vi "test Correct Subaddresses In Log.vi"(8 "error in (no error)":errorcluster, 11 "TestCase in":refnum<class "Logging Loopback.lvclass">) -> (0 "error out":errorcluster, 3 "TestCase out":refnum<class "Logging Loopback.lvclass">)   [LabVIEW 2020, in "Logging Loopback.lvclass"]
uses:
  Logging Loopback.lvclass
  Logging Loopback.lvclass/Logging Loopback.ctl
  6070ecc1-7a7f-4aba-84f3-8f274e3c644e.vi
  e19d9c75-8616-4056-a7e1-33fbf9884e17.vi
  <vilib>/WebDAVClient/Advanced/Get Buffer.vi
  <vilib>/addons/_JKI Toolkits/VI Tester/TestCase.llb/TestCase.lvclass
  <vilib>/WebDAVClient/NI_WebDAV.lvlib
  C:/Program Files (x86)/National Instruments/LabVIEW 2020/vi.lib/addons/_JKI Toolkits/VI Tester/TestCase.llb/TestCase.lvclass
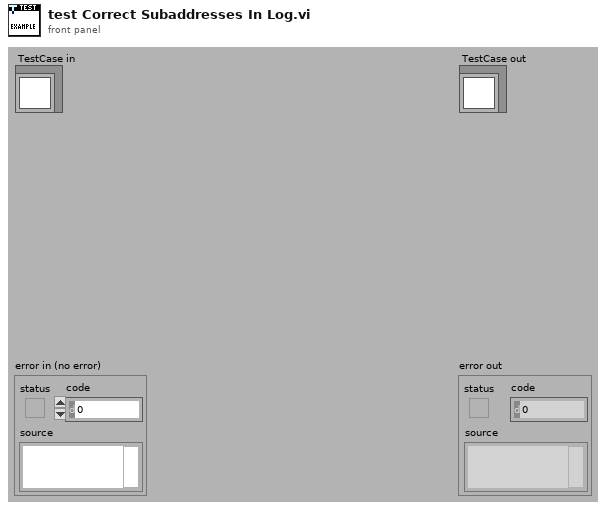
[diagram p1: front panel]
types:
  T1 = typedef "NI_WebDAV.lvlib/SessionHandle.ctl" = refnum<k1>
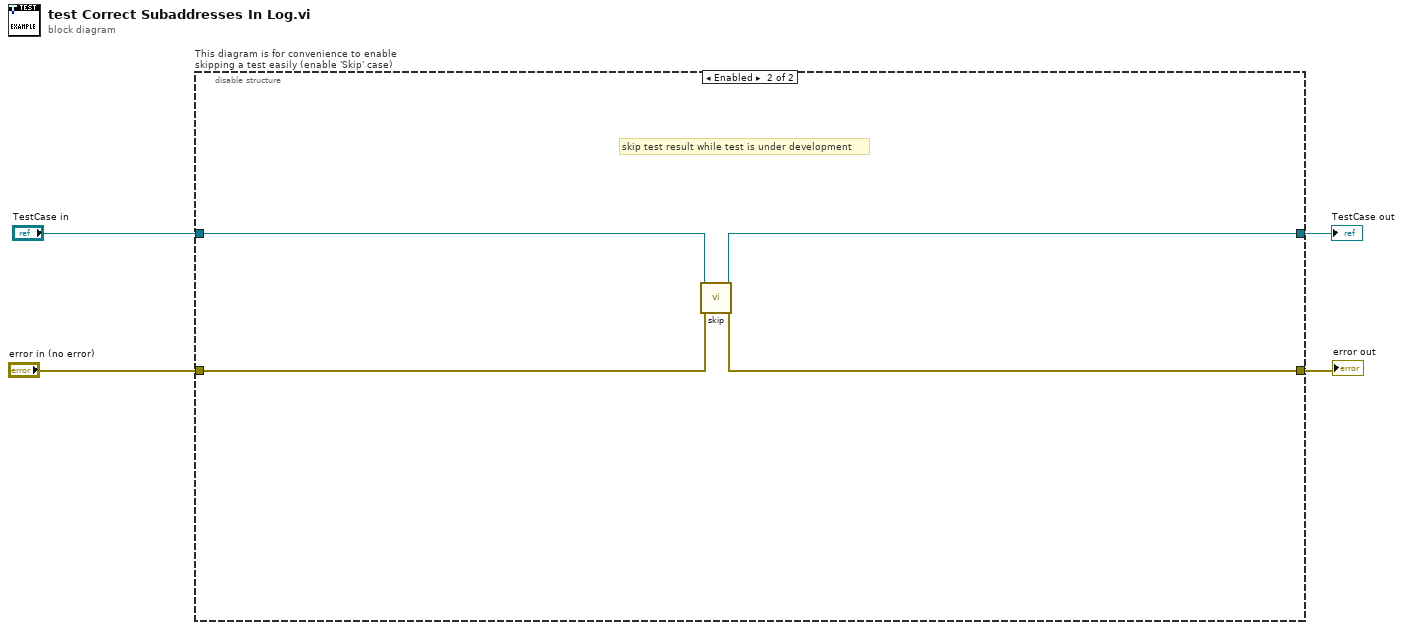
[diagram p0: block diagram]
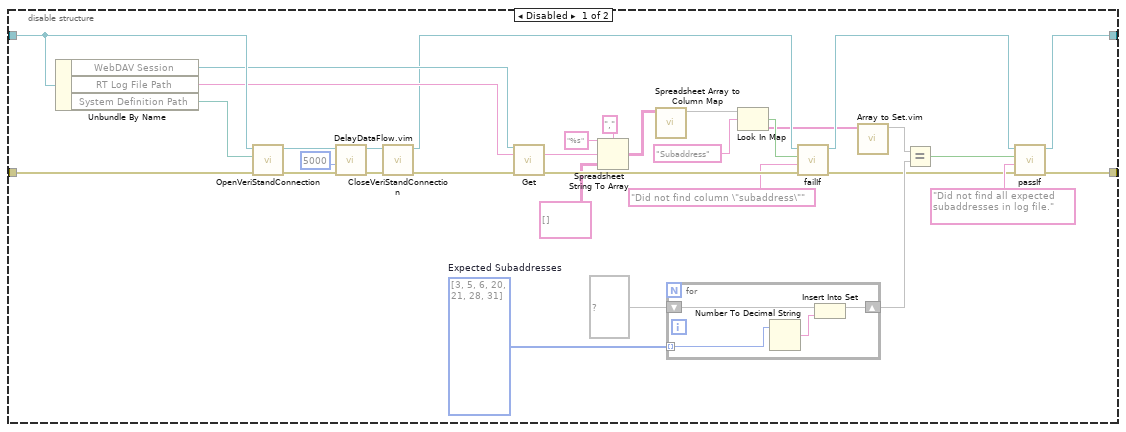
[diagram p2: hidden frame]
diagram:
  n1 = disable-structure "This diagram is for convenience to enable skipping a test easily (enable 'Skip' case)" shown="Enabled" {
    disable-tunnel: "TestCase in" -> [w33 w44]
    disable-tunnel: [w16 w42] -> w1
    disable-tunnel: [w17 w43] -> w3
    disable-tunnel: "error in (no error)" -> [w36 w41]
    frame Disabled {
      w5 = i32[] [3, 5, 6, 20, 21, 28, 31]  # Expected Subaddresses
      n2 = Unbundle By Name(w33) -> ("WebDAV Session"=w27:T1, "RT Log File Path"=w26:string, "System Definition Path"=w34:path)
      n3 = call-dynamic "OpenVeriStandConnection.vi"("error in (no error)"=w36, "System Definition File"=w34, "VeriStand Test Case in"=w33) -> ("error out"=w35:errorcluster, "VeriStand Test Case out"=w30:refnum<class "Logging Loopback.lvclass">)  [unwired: 6 in, 1 out]
      n4 = call "DelayDataFlow.vim"("value in"=w35, "milliseconds to wait"=u32 5000) -> ("value out"=w32:errorcluster)  [unwired: 2 in, 1 out]
      n5 = call-dynamic "CloseVeriStandConnection.vi"("error in (no error)"=w32, "VeriStand Test Case in"=w30) -> ("error out"=w29:errorcluster, "VeriStand Test Case out"=w10:refnum<class "Logging Loopback.lvclass">)  [unwired: 8 in]
      n6 = call-poly <vilib>:"Get.vi"("session handle"=w27, "relative uri"=w26, "error in (no error)"=w29) -> ("data"=w25:string, "error out"=w28:errorcluster)  [unwired: 10 in, 1 out]
      n7 = Spreadsheet String To Array(delimiter (Tab)=",", format string="%s", spreadsheet string=w25, array type (2D Dbl)=string[][] []) -> (array=w21:string[][])
      n8 = call "Spreadsheet Array to Column Map.vi"("array"=w21) -> ("map"=w20:map{string, string[]})  [unwired: 10 in]
      n9 = for {
        shift-right: [w39] -> w14
        shift-left: set{string} {} ("set in") -> [w40]
        tunnel: w5 -> [w37] mode=indexing
        n10 = Number To Decimal String(number=w37) -> (decimal integer string=w38:string)  [unwired: 1 in]
        n11 = Insert Into Set(10:w38, 11:w40) -> (3:w39:set{string})  [unwired: 1 out]
      }
      n12 = Look In Map(map=w20, key="Subaddress") -> (key not found?=w8:bool, value=w6:string[])  [unwired: 1 in]
      n13 = call-dynamic "failIf.vi"("error in (no error)"=w28, "message (\"\")"="Did not find column \"subaddress\"" ("message (\"\")"), "fail"=w8, "TestCase in"=w10) -> ("error out"=w11:errorcluster, "TestCase out"=w9:refnum<class "Logging Loopback.lvclass">)  [unwired: 6 in]
      n14 = call "Array to Set.vim"("array"=w6) -> ("set"=w15:set{string})  [unwired: 10 in]
      n15 = Equal?(x=w15, y=w14) -> (x = y?=w13:bool)
      n16 = call-dynamic "passIf.vi"("error in (no error)"=w11, "message (\"\")"="Did not find all expected subaddresses in log file." ("message (\"\")"), "pass"=w13, "TestCase in"=w9) -> ("error out"=w17:errorcluster, "TestCase out"=w16:refnum<class "Logging Loopback.lvclass">)  [unwired: 6 in]
    }
    frame Enabled {
      # "skip test result while test is under development"
      n17 = call <vilib>:"skip.vi"("error in (no error)"=w41, "TestCase in"=w44) -> ("error out"=w43:errorcluster, "TestCase out"=w42:refnum<class "Logging Loopback.lvclass">)  [unwired: 8 in]
    }
  }
  "error out" <- w3
  "TestCase out" <- w1
